vi "unwrap2D_main.vi"   [LabVIEW 2015]
types:
  T1 = typedef "NI_Matrix.lvlib/RealMatrix.ctl" = dbl[][]
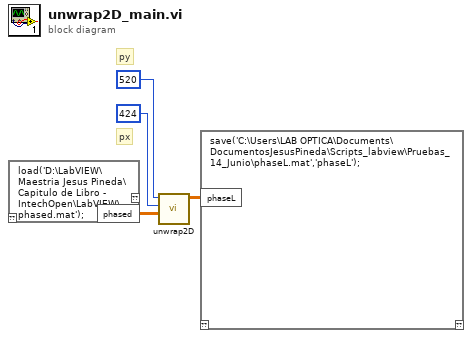
[diagram p0: block diagram]
diagram:
  # "py"
  # "px"
  n1 = script code="load('D:\\LabVIEW\\Maestria Jesus Pineda\\Capitulo de Libro - IntechOpen\\LabVIEW\\phased.mat');"() -> ("phased"=w4:dbl[][])  [unwired: 1 in, 1 out]
  n2 = call "unwrap2D.vi"("Array"=w4, "Numeric 2"=424, "Numeric"=520) -> ("A + B"=w3:T1)  [unwired: 8 in]
  n3 = script code="save('C:\\Users\\LAB OPTICA\\Documents\\DocumentosJesusPineda\\Scripts_labview\\Pruebas_14_Junio\\phaseL.mat','phaseL');"("phaseL"=w3) -> ()  [unwired: 1 in, 1 out]
